vi "CVT I32 StaticWrite.vi"(3 "error in (no error)":errorcluster, 4 "Value":i32, 5 "Tag Name":string) -> (0 "error out":errorcluster)   [LabVIEW 2014, in "QwaveSys Raspberry Pi Library.lvlib"]
uses:
  _SubVIs/TypeDefs/cvt_MemBlock Methods.ctl
  _SubVIs/TypeDefs/cvt_TagList Methods.ctl
  QwaveSys Raspberry Pi Library.lvlib
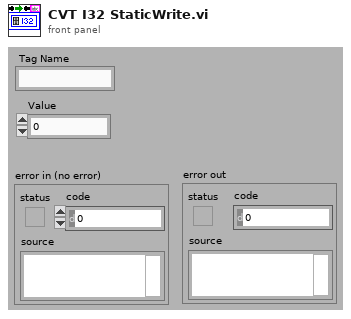
[diagram p1: front panel]
types:
  T1 = typedef "QwaveSys Raspberry Pi Library.lvlib/cvt_MemBlock Methods.ctl" = enum16{"init", "read", "readall", "write"}
  T2 = typedef "QwaveSys Raspberry Pi Library.lvlib/cvt_TagList Methods.ctl" = enum16{"init", "getindex", "getdesc", "getlist"}
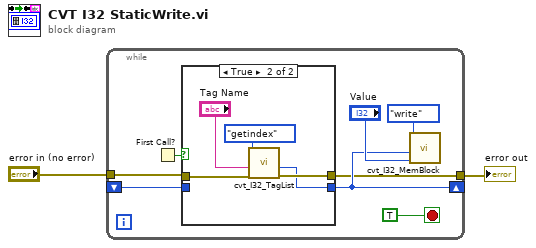
[diagram p0: block diagram]
diagram:
  n1 = while {
    shift-right: [w5] -> _
    shift-left: _ -> [w7]
    tunnel: [w3] -> w2
    tunnel: "error in (no error)" -> [w6]
    stop <- TRUE stop-if-true
    n2 = First Call?() -> (First Call?: T/F=w8:bool)
    n3 = case shown="True" w8 {
      tunnel: [w12 w14] -> w5
      tunnel: w7 -> [w12 _]
      tunnel: w6 -> [w11 w16]
      tunnel: [w11 w15] -> w3
      frame False {
      }
      frame True {
        n4 = call "cvt_I32_TagList.vi"("error in (no error)"=w16, "Tag Name"="Tag Name", "Method"=cvt_TagList_Methods."getindex") -> ("error out"=w15:errorcluster, "Index"=w14:i32)  [unwired: 1 in, 6 out]
      }
    }
    n5 = call "cvt_I32_MemBlock.vi"("Value"="Value", "Index"=w5, "Method"=cvt_MemBlock_Methods."write") -> ()  [unwired: 2 in, 7 out]
  }
  "error out" <- w2
